vi "RSZVB Save Recall Ripple Limit.vi"(7 "File Name":string, 8 "error in (no error)":errorcluster {"code" format="%.0x"}, 9 "Trace Name":string, 10 "Operation to be Performed (0: Save)":i32(ring) items=["Save", "Recall"], 11 "VISA session":refnum<visa-resource-name>) -> (0 "error out":errorcluster {"code" format="%.0x"}, 3 "dup VISA session":refnum<visa-resource-name>)   [LabVIEW 2011]
doc: "This VI saves or recalls the ripple limits associated with a specified trace.\n\nRemote-control command(s):\nMMEMory:LOAD:RIPPle 'Trc_name','file_name'\nMMEMory:STORe:RIPPle 'Trc_name','file_name'"
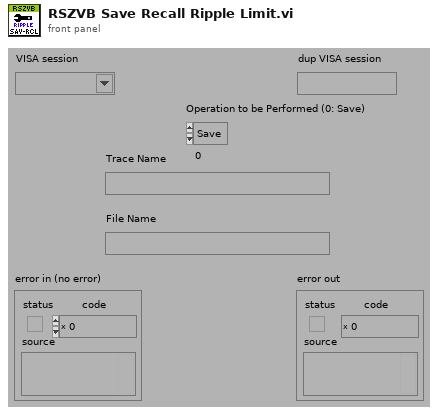
[diagram p1: front panel]
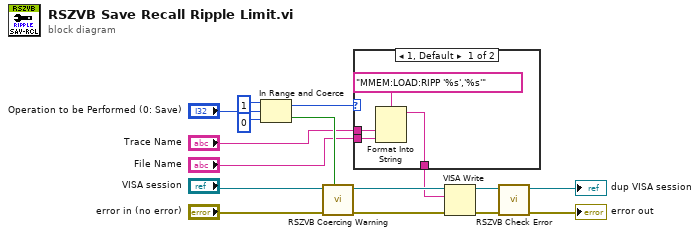
[diagram p0: block diagram]
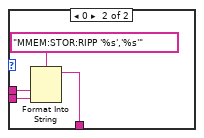
[diagram p2: hidden frame]
diagram:
  n1 = In Range and Coerce(upper limit=1, x="Operation to be Performed (0: Save)", lower limit=0) -> (coerced(x)=w1:i32, In Range?=w4:bool)
  n2 = call "RSZVB Coercing Warning.vi"("In Range?"=w4, "error in (no error)"="error in (no error)", "VISA session"="VISA session") -> ("error out"=w15:errorcluster, "dup VISA session"=w16:refnum<visa-resource-name>)  [unwired: 7 in]
  n3 = case shown="1, Default" w1 {
    tunnel: [w19 w23] -> w12
    tunnel: "Trace Name" -> [w18 w22]
    tunnel: "File Name" -> [w17 w21]
    frame 1, Default {
      n4 = Format Into String(format string="MMEM:LOAD:RIPP '%s','%s'", w18, w17) -> (resulting string=w19:string)  [unwired: 2 in, 1 out]
    }
    frame 0 {
      n5 = Format Into String(format string="MMEM:STOR:RIPP '%s','%s'", w22, w21) -> (resulting string=w23:string)  [unwired: 2 in, 1 out]
    }
  }
  n6 = VISA Write(VISA resource name=w16, write buffer=w12, error in (no error)=w15) -> (VISA resource name out=w13:refnum<visa-resource-name>, error out=w14:errorcluster)  [unwired: 1 out]
  n7 = call "RSZVB Check Error.vi"("error in (no error)"=w14, "VISA session"=w13) -> ("error out"=→"error out":errorcluster, "dup VISA session"=→"dup VISA session":refnum<visa-resource-name>)  [unwired: 8 in]
